vi "Map Structure to [0,1).vi"(11 "Structure":T1={"Structure ID"="Batch3_1", "Lattice vector a"=[6.48, 0.0, 0.0], "Lattice vector b"=[0.0, 6.48, 0.0], "Lattice vector c"=[0.0, 0.0, 31.06], "Atoms Array"=[{"Atom Name"="Cd", "Positions (Direct)"=[[0.0, 0.0, 0.00272], [0.5, 0.5, 0.00272], [0.5, 0.0, 0.110479], [0.0, 0.5, 0.110479], [0.0, 0.0, 0.218487], [0.5, 0.5, 0.218487], [0.5, 0.0, 0.32654], [0.0, 0.5, 0.32654], [0.25, 0.25, 0.427635], [0.75, 0.75, 0.427635], [0.0, 0.0, 0.570345], [0.5, 0.5, 0.570345], [0.5, 0.0, 0.679049], [0.0, 0.5, 0.679049], [0.0, 0.0, 0.786972], [0.5, 0.5, 0.786972], [0.5, 0.0, 0.894944], [0.0, 0.5, 0.894944]], "Positions (Cartesian)"=[[0.0, 0.0, 0.08448320000000001], [3.24, 3.24, 0.08448320000000001], [3.24, 0.0, 3.4314777399999996], [0.0, 3.24, 3.4314777399999996], [0.0, 0.0, 6.7862062199999995], [3.24, 3.24, 6.7862062199999995], [3.24, 0.0, 10.142332399999999], [0.0, 3.24, 10.142332399999999], [1.62, 1.62, 13.282343099999999], [4.86, 4.86, 13.282343099999999], [0.0, 0.0, 17.7149157], [3.24, 3.24, 17.7149157], [3.24, 0.0, 21.09126194], [0.0, 3.24, 21.09126194], [0.0, 0.0, 24.44335032], [3.24, 3.24, 24.44335032], [3.24, 0.0, 27.796960639999998], [0.0, 3.24, 27.796960639999998]]}, {"Atom Name"="Te", "Positions (Direct)"=[[0.25, 0.25, 0.055996], [0.75, 0.75, 0.055996], [0.75, 0.25, 0.163889], [0.25, 0.75, 0.163889], [0.25, 0.25, 0.271952], [0.75, 0.75, 0.271952], [0.75, 0.25, 0.383704], [0.25, 0.75, 0.383704], [0.0, 0.0, 0.483915], [0.5, 0.5, 0.483915], [0.25, 0.25, 0.623906], [0.75, 0.75, 0.623906], [0.75, 0.25, 0.732362], [0.25, 0.75, 0.732362], [0.25, 0.25, 0.840344], [0.75, 0.75, 0.840344], [0.75, 0.25, 0.948333], [0.25, 0.75, 0.948333]], "Positions (Cartesian)"=[[1.62, 1.62, 1.73923576], [4.86, 4.86, 1.73923576], [4.86, 1.62, 5.09039234], [1.62, 4.86, 5.09039234], [1.62, 1.62, 8.44682912], [4.86, 4.86, 8.44682912], [4.86, 1.62, 11.91784624], [1.62, 4.86, 11.91784624], [0.0, 0.0, 15.030399899999999], [3.24, 3.24, 15.030399899999999], [1.62, 1.62, 19.37852036], [4.86, 4.86, 19.37852036], [4.86, 1.62, 22.747163719999996], [1.62, 4.86, 22.747163719999996], [1.62, 1.62, 26.10108464], [4.86, 4.86, 26.10108464], [4.86, 1.62, 29.45522298], [1.62, 4.86, 29.45522298]]}], "# of atoms"=36}) -> (3 "Structure mapped to [0,1)":T1={"Structure ID"="Batch3_1", "Lattice vector a"=[6.48, 0.0, 0.0], "Lattice vector b"=[0.0, 6.48, 0.0], "Lattice vector c"=[0.0, 0.0, 31.06], "Atoms Array"=[{"Atom Name"="Cd", "Positions (Direct)"=[[0.0, 0.0, 0.00272], [0.5, 0.5, 0.00272], [0.5, 0.0, 0.110479], [0.0, 0.5, 0.110479], [0.0, 0.0, 0.218487], [0.5, 0.5, 0.218487], [0.5, 0.0, 0.32654], [0.0, 0.5, 0.32654], [0.25, 0.25, 0.427635], [0.75, 0.75, 0.427635], [0.0, 0.0, 0.570345], [0.5, 0.5, 0.570345], [0.5, 0.0, 0.679049], [0.0, 0.5, 0.679049], [0.0, 0.0, 0.786972], [0.5, 0.5, 0.786972], [0.5, 0.0, 0.894944], [0.0, 0.5, 0.894944]], "Positions (Cartesian)"=[[0.0, 0.0, 0.08448320000000001], [3.24, 3.24, 0.08448320000000001], [3.24, 0.0, 3.4314777399999996], [0.0, 3.24, 3.4314777399999996], [0.0, 0.0, 6.7862062199999995], [3.24, 3.24, 6.7862062199999995], [3.24, 0.0, 10.142332399999999], [0.0, 3.24, 10.142332399999999], [1.62, 1.62, 13.282343099999999], [4.86, 4.86, 13.282343099999999], [0.0, 0.0, 17.7149157], [3.24, 3.24, 17.7149157], [3.24, 0.0, 21.09126194], [0.0, 3.24, 21.09126194], [0.0, 0.0, 24.44335032], [3.24, 3.24, 24.44335032], [3.24, 0.0, 27.796960639999998], [0.0, 3.24, 27.796960639999998]]}, {"Atom Name"="Te", "Positions (Direct)"=[[0.25, 0.25, 0.055996], [0.75, 0.75, 0.055996], [0.75, 0.25, 0.163889], [0.25, 0.75, 0.163889], [0.25, 0.25, 0.271952], [0.75, 0.75, 0.271952], [0.75, 0.25, 0.383704], [0.25, 0.75, 0.383704], [0.0, 0.0, 0.483915], [0.5, 0.5, 0.483915], [0.25, 0.25, 0.623906], [0.75, 0.75, 0.623906], [0.75, 0.25, 0.732362], [0.25, 0.75, 0.732362], [0.25, 0.25, 0.840344], [0.75, 0.75, 0.840344], [0.75, 0.25, 0.948333], [0.25, 0.75, 0.948333]], "Positions (Cartesian)"=[[1.62, 1.62, 1.73923576], [4.86, 4.86, 1.73923576], [4.86, 1.62, 5.09039234], [1.62, 4.86, 5.09039234], [1.62, 1.62, 8.44682912], [4.86, 4.86, 8.44682912], [4.86, 1.62, 11.91784624], [1.62, 4.86, 11.91784624], [0.0, 0.0, 15.030399899999999], [3.24, 3.24, 15.030399899999999], [1.62, 1.62, 19.37852036], [4.86, 4.86, 19.37852036], [4.86, 1.62, 22.747163719999996], [1.62, 4.86, 22.747163719999996], [1.62, 1.62, 26.10108464], [4.86, 4.86, 26.10108464], [4.86, 1.62, 29.45522298], [1.62, 4.86, 29.45522298]]}], "# of atoms"=36})   [LabVIEW 2010]
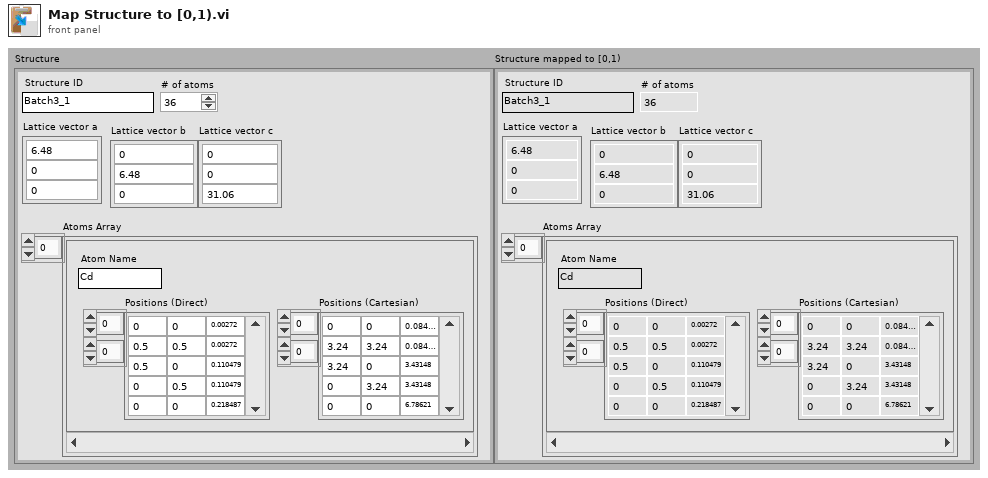
[diagram p1: front panel]
types:
  T1 = cluster{"Structure ID":string, "Lattice vector a":dbl[], "Lattice vector b":dbl[], "Lattice vector c":dbl[], "Atoms Array":cluster{"Atom Name":string, "Positions (Direct)":dbl[][], "Positions (Cartesian)":dbl[][]}[], "# of atoms":i32}
  T2 = cluster{"Atom Name":string, "Positions (Direct)":dbl[][], "Positions (Cartesian)":dbl[][]}[]
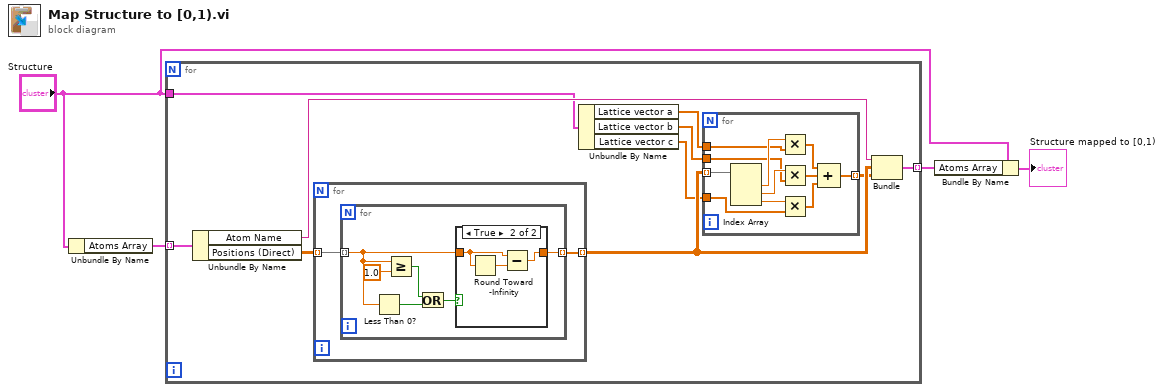
[diagram p0: block diagram]
diagram:
  n1 = Unbundle By Name("Structure") -> ("Atoms Array"=w4:T2)
  n2 = for {
    tunnel: w4 -> [w14] mode=indexing
    tunnel: "Structure" -> [w9]
    tunnel: [w11] -> w1 mode=indexing
    n3 = Unbundle By Name(w14) -> ("Atom Name"=w12:string, "Positions (Direct)"=w13:dbl[][])
    n4 = for {
      tunnel: w13 -> [w27] mode=indexing
      tunnel: [w26] -> w10 mode=indexing
      n5 = for {
        tunnel: w27 -> [w32] mode=indexing
        tunnel: [w31] -> w26 mode=indexing
        n6 = Less Than 0?(x=w32) -> (x < 0?=w29:bool)
        n7 = Greater Or Equal?(x=w32, y=1.0) -> (x >= y?=w30:bool)
        n8 = Or(x=w30, y=w29) -> (x .or. y?=w28:bool)
        n9 = case shown="True" w28 {
          tunnel: w32 -> [w34 w35]
          tunnel: [w34 w36] -> w31
          frame False {
          }
          frame True {
            n10 = Round Toward -Infinity(1:w35) -> (0:w37:dbl)
            n11 = Subtract(x=w35, y=w37) -> (x-y=w36:dbl)
          }
        }
      }
    }
    n12 = Unbundle By Name(w9) -> ("Lattice vector a"=w8:dbl[], "Lattice vector b"=w7:dbl[], "Lattice vector c"=w6:dbl[])
    n13 = for {
      tunnel: w10 -> [w25] mode=indexing
      tunnel: w8 -> [w23]
      tunnel: w7 -> [w21]
      tunnel: w6 -> [w19]
      tunnel: [w15] -> w5 mode=indexing
      n14 = Index Array(array=w25) -> (element #1=w24:dbl, element #2=w22:dbl, element #3=w20:dbl)  [unwired: 3 in]
      n15 = Multiply(x=w24, y=w23) -> (x*y=w18:dbl[])
      n16 = Multiply(x=w22, y=w21) -> (x*y=w17:dbl[])
      n17 = Multiply(x=w20, y=w19) -> (x*y=w16:dbl[])
      n18 = Compound Arithmetic op=ADD(w18, w17, w16) -> (w15:dbl[])
    }
    n19 = Bundle("Atom Name"=w12, w10, w5) -> (w11:cluster{"Atom Name":string, dbl[][], dbl[][]})  [unwired: 1 in]
  }
  n20 = Bundle By Name(cluster="Structure", "Atoms Array"=w1) -> (→"Structure mapped to [0,1)":T1)
